vi "Practica_medicion_remota2_ESCRITURA[2].vi"() -> ()   [LabVIEW 2020]
uses:
  <vilib>/httpClient/PUTBuffer.vi
  <vilib>/httpClient/LabVIEWHTTPClient.lvlib
panel:
  out "body":string
  out "headers":string
  in  "stop":bool
  out "error out":errorcluster
  in  "Acondicionamiento [mA]":dbl(knob) scale=0.0..10.0
  in  "Boolean":bool
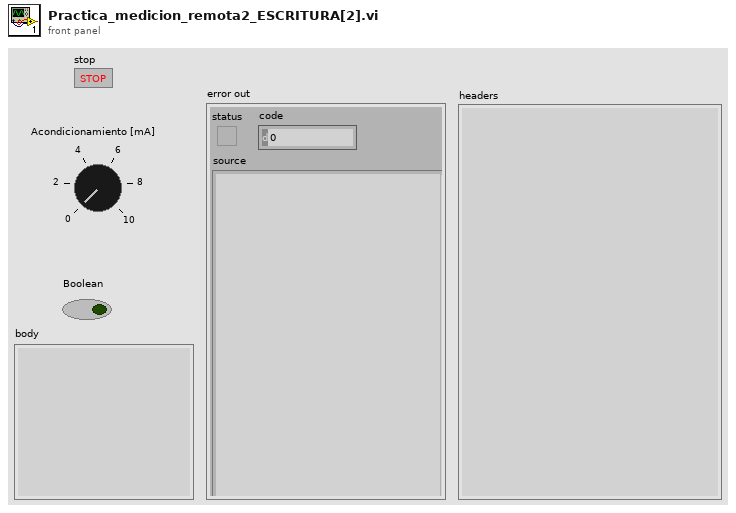
[diagram p1: front panel]
types:
  T1 = cluster{"Rele":bool, "Hora":string, "Data":string, "Acondicionamiento":dbl}
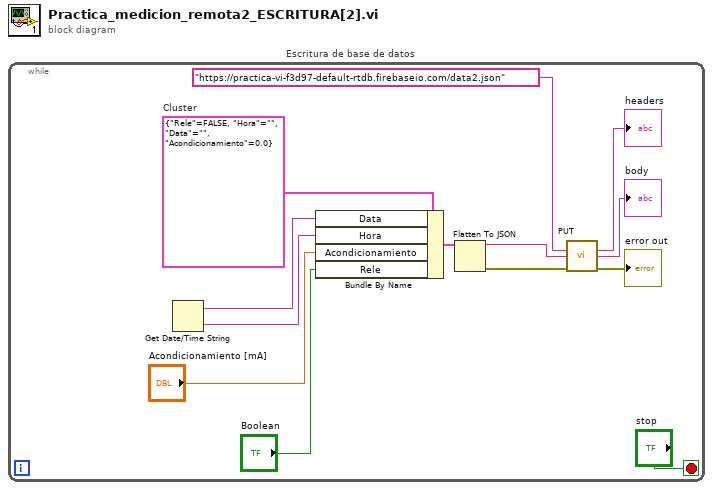
[diagram p0: block diagram]
diagram:
  n1 = while "Escritura de base de datos" {
    stop <- "stop" stop-if-true
    w1 = T1 {"Rele"=FALSE, "Hora"="", "Data"="", "Acondicionamiento"=0.0}  # Cluster
    n2 = Get Date/Time String() -> (date string=w5:string, time string=w4:string)  [unwired: 3 in]
    n3 = Bundle By Name "Bundle By Name"(cluster=w1, "Data"=w5, "Hora"=w4, "Acondicionamiento"="Acondicionamiento [mA]", "Rele"="Boolean") -> (w12:T1)
    n4 = Flatten To JSON(anything=w12) -> (JSON string=w11:string, 11:w10:errorcluster)  [unwired: 2 in]
    n5 = call-poly <vilib>:"PUT.vi"("url"="https://practica-vi-f3d97-default-rtdb.firebaseio.com/data2.json", "buffer"=w11, "error in (no error)"=w10) -> ("headers"=→"headers":string, "body"=→"body":string, "error out"=→"error out":errorcluster)  [unwired: 9 in, 1 out]
  }
